vi "hash.vi"() -> ()   [LabVIEW 2010]
panel:
  in  "String":string
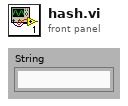
[diagram p1: front panel]
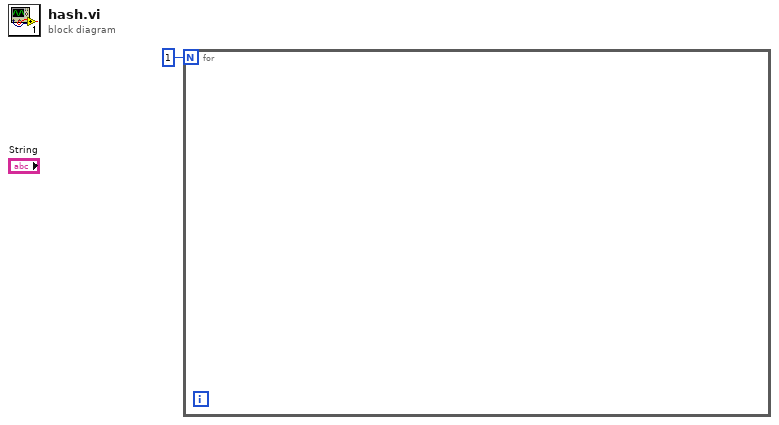
[diagram p0: block diagram]
diagram:
  n1 = for {
    N: 1 -> [_]
  }
